vi "PolyLaguerre.vi"(1 "n":i32) -> (0 "Ln":dbl[](array[numeric]))   [LabVIEW 2020, in "NI_AALPro.lvlib"]
uses:
  NI_AALPro.lvlib
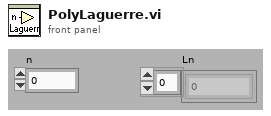
[diagram p1: front panel]
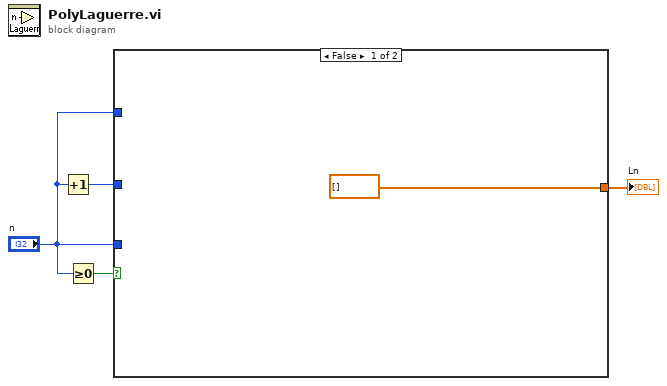
[diagram p0: block diagram]
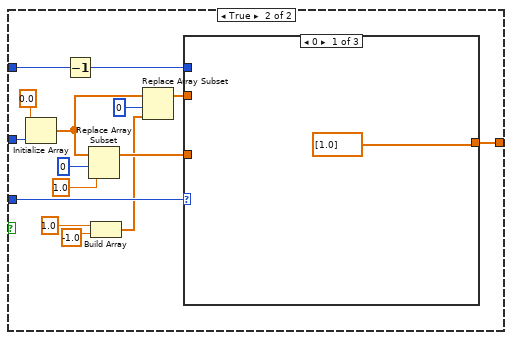
[diagram p2: hidden frame]
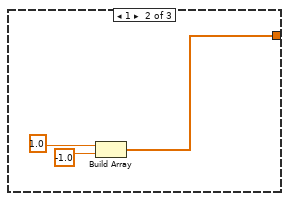
[diagram p3: hidden frame]
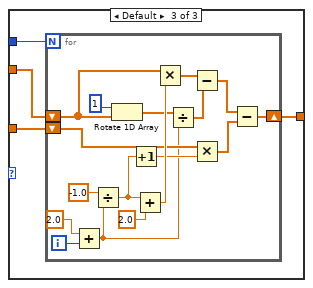
[diagram p4: hidden frame]
diagram:
  n1 = Increment(x="n") -> (x+1=w3:i32)
  n2 = Greater Or Equal To 0?(x="n") -> (x >= 0?=w4:bool)
  n3 = case shown="False" w4 {
    tunnel: "n" -> [_ w20]
    tunnel: w3 -> [_ w14]
    tunnel: "n" -> [_ w12]
    tunnel: [dbl[] [] ("Tn(x)") w13] -> w1
    frame False {
    }
    frame True {
      n4 = Initialize Array(0.0 ("element"), w14) -> (w10:dbl[])
      n5 = Decrement(x=w12) -> (x-1=w11:i32)
      n6 = Replace Array Subset(array=w10, new element=1.0 ("new element/subarray"), index=0) -> (w9:dbl[])
      n7 = Build Array(1.0 ("element"), -1.0 ("element")) -> (w7:dbl[])
      n8 = Replace Array Subset(array=w10, new element=w7, index=0) -> (w15:dbl[])
      n9 = case shown="0" w20 {
        tunnel: w15 -> [_ _ w28]
        tunnel: w9 -> [_ _ w27]
        tunnel: w11 -> [_ _ w26]
        tunnel: [dbl[] [1.0] ("Tn(x)") w23 w25] -> w13
        frame 0 {
        }
        frame 1 {
          n10 = Build Array(1.0 ("element"), -1.0 ("element")) -> (w23:dbl[])
        }
        frame Default {
          n11 = for {
            N: w26 -> [_]
            shift-right: [w34] -> w25
            shift-left: w28 -> [w41]
            shift-left: w27 -> [w35]
            i -> [w44]
            n12 = Add(x=2.0, y=w44) -> (x+y=w31:dbl)
            n13 = Divide(x=-1.0, y=w31) -> (x/y=w30:dbl)
            n14 = Rotate 1D Array(1:w41, 2:1 ("n")) -> (0:w38:dbl[])
            n15 = Increment(x=w30) -> (x+1=w36:dbl)
            n16 = Add(x=w30, y=2.0) -> (x+y=w40:dbl)
            n17 = Multiply(x=w41, y=w40) -> (x*y=w39:dbl[])
            n18 = Divide(x=w38, y=w31) -> (x/y=w37:dbl[])
            n19 = Subtract(x=w39, y=w37) -> (x-y=w33:dbl[])
            n20 = Multiply(x=w35, y=w36) -> (x*y=w32:dbl[])
            n21 = Subtract(x=w33, y=w32) -> (x-y=w34:dbl[])
          }
        }
      }
    }
  }
  "Ln" <- w1
